vi "Set plotnames test.vi"() -> ()   [LabVIEW 2018]
panel:
  in  "플롯 이름":string[](array[string])
  out "XY 그래프":cluster{"X":dbl, "Y":dbl}[](graph)
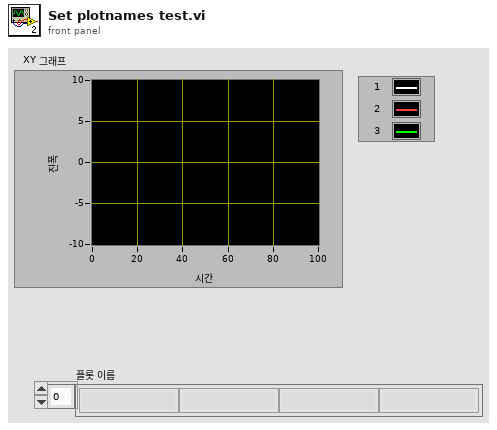
[diagram p1: front panel]
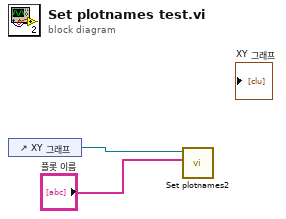
[diagram p0: block diagram]
diagram:
  n1 = control-ref of="XY 그래프"() -> (w2:refnum<vi>)
  n2 = call "Set plotnames2.vi"("플롯 이름"="플롯 이름", "그래프 참조"=w2) -> ()  [unwired: 9 in, 1 out]
